vi "Configure Clock.vi"(7 "Interpolation":u16=1, 8 "error in (no error)":errorcluster, 9 "Rate of External Sample Clock (MHz)":u16=60 min=60 max=100 step=1, 10 "Clock Select":u32, 11 "FPGA VI Reference In":refnum<k20>) -> (0 "error out":errorcluster, 1 "User Command Error":u16, 2 "Successfully Configured?":bool, 3 "FPGA VI Reference Out":refnum<k20>, 4 "Sampling Rate":dbl)   [LabVIEW 2020]
uses:
  Controls/User Command.ctl
  <vilib>/Utility/error.llb/Error Cluster From Error Code.vi
  <vilib>/rvi/errors/niLvFpgaAdjustHostInterfaceError.vi
  <vilib>/rvi/interface/nirviReadWriteControl/nirviReadWriteControl.xnode
  NiFpgaLv.dll
  <vilib>/rvi/interface/Simulation/niFpgaSimulationCallBeginRW.vi
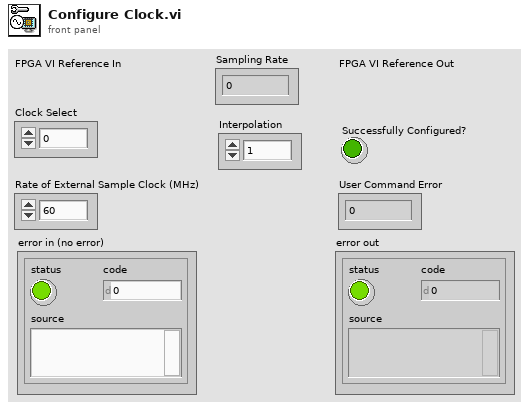
[diagram p1: front panel]
types:
  T1 = typedef "User Command.ctl" = u16
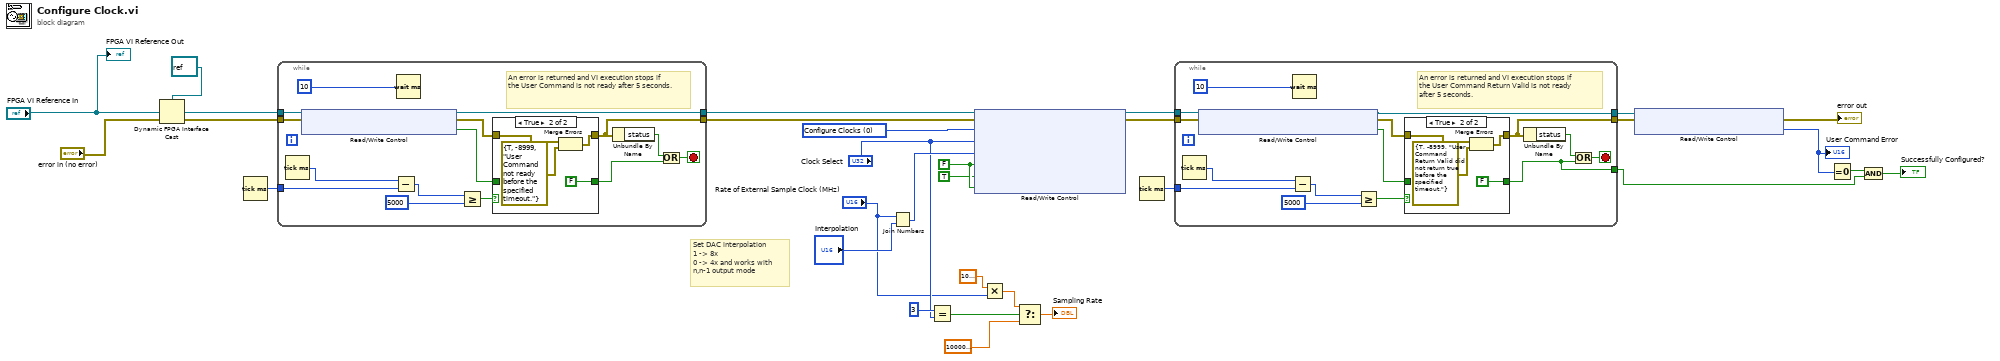
[diagram p0: block diagram]
diagram:
  w24 = FALSE ("IO Module\\User Command Valid")
  w25 = T1 0 items=["Reintialize"=65535, "Get CLIP Version"=65520, "SPI Write Verify"=65026, "SPI Write"=65025, "SPI Read"=65024, "I2C Write"=64769, "I2C Read"=64768, "Configure Clocks"=0]
  # "Set DAC interpolation \n1 -> 8x\n0 -> 4x and works with \nn,n-1 output mode"
  n1 = Dynamic FPGA Interface Cast(Session In=refnum<k20> refnum ("Refnum in"), Type="FPGA VI Reference In") -> (Session Out=w28:refnum<k20>)
  n2 = Tick Count (ms)() -> (millisecond timer value=w27:u32)
  n3 = while {
    tunnel: "error in (no error)" -> [w38]
    tunnel: [w42] -> w20
    tunnel: w28 -> [w37]
    tunnel: w27 -> [w33]
    tunnel: [w31] -> w26
    stop <- w40 stop-if-true
    # "An error is returned and VI execution stops if the User Command is not ready after 5 seconds."
    n4 = Tick Count (ms)() -> (millisecond timer value=w34:u32)
    n5 = xnode "Read/Write Control"("FPGA VI Reference In"=w37, "error in"=w38) -> ("FPGA VI Reference Out"=w31:refnum<k20>, "error out"=w35:errorcluster, "IO Module\\User Command Ready"=w36:bool)
    n6 = Subtract(x=w34, y=w33) -> (x-y=w32:u32)
    n7 = Wait (ms)(milliseconds to wait=u32 10) -> ()  [unwired: 1 out]
    n8 = Greater Or Equal?(x=w32, y=u32 5000) -> (x >= y?=w43:bool)
    n9 = case shown="True" w43 {
      tunnel: [w47 FALSE ("Configured?")] -> w39
      tunnel: w36 -> [w47 _]
      tunnel: [w46 w50] -> w42
      tunnel: w35 -> [w46 w48]
      frame False {
      }
      frame True {
        n10 = Merge Errors(w48, errorcluster {"status"=TRUE, "code"=-8999, "source"="User Command not ready before the specified timeout."} ("error in")) -> (w50:errorcluster)
      }
    }
    n11 = Unbundle By Name(w42) -> ("status"=w41:bool)
    n12 = Or(x=w41, y=w39) -> (x .or. y?=w40:bool)
  }
  n13 = Join Numbers(hi="Rate of External Sample Clock (MHz)", lo="Interpolation") -> ((hi.lo)=w21:u32)
  n14 = Equal?(x=u16 3, y="Clock Select") -> (x = y?=w8:bool)
  n15 = xnode "Read/Write Control"("FPGA VI Reference In"=w26, "error in"=w20, "IO Module\\User Command"=w25, "IO Module\\User Command Arg 0"="Clock Select", "IO Module\\User Command Arg 1"=w21, "IO Module\\User Command Valid"=w24, "IO Module\\User Command Valid"=TRUE ("IO Module\\User Command Valid"), "IO Module\\User Command Valid"=w24) -> ("FPGA VI Reference Out"=w18:refnum<k20>, "error out"=w17:errorcluster)
  n16 = Multiply(x=1000000.0 ("Sample Rate"), y="Rate of External Sample Clock (MHz)") -> (x*y=w5:dbl)
  n17 = Select(t=w5, s=w8, f=100000000.0 ("Sample Rate")) -> (s? t:f=→"Sampling Rate":dbl)
  n18 = Tick Count (ms)() -> (millisecond timer value=w19:u32)
  n19 = while {
    tunnel: w17 -> [w60]
    tunnel: [w63] -> w11
    tunnel: w18 -> [w59]
    tunnel: w19 -> [w55]
    tunnel: [w53] -> w16
    tunnel: [w52] -> w13
    stop <- w61 stop-if-true
    # "An error is returned and VI execution stops if the User Command Return Valid is not ready after 5 seconds."
    n20 = Tick Count (ms)() -> (millisecond timer value=w56:u32)
    n21 = xnode "Read/Write Control"("FPGA VI Reference In"=w59, "error in"=w60) -> ("FPGA VI Reference Out"=w53:refnum<k20>, "error out"=w57:errorcluster, "IO Module\\User Command Return Valid"=w58:bool)
    n22 = Subtract(x=w56, y=w55) -> (x-y=w54:u32)
    n23 = Wait (ms)(milliseconds to wait=u32 10) -> ()  [unwired: 1 out]
    n24 = Greater Or Equal?(x=w54, y=u32 5000) -> (x >= y?=w64:bool)
    n25 = case shown="True" w64 {
      tunnel: [w68 FALSE ("Configured?")] -> w52
      tunnel: w58 -> [w68 _]
      tunnel: [w67 w71] -> w63
      tunnel: w57 -> [w67 w69]
      frame False {
      }
      frame True {
        n26 = Merge Errors(w69, errorcluster {"status"=TRUE, "code"=-8999, "source"="User Command Return Valid did not return true before the specified timeout."} ("error in")) -> (w71:errorcluster)
      }
    }
    n27 = Unbundle By Name(w63) -> ("status"=w62:bool)
    n28 = Or(x=w62, y=w52) -> (x .or. y?=w61:bool)
  }
  n29 = xnode "Read/Write Control"("FPGA VI Reference In"=w16, "error in"=w11) -> ("error out"=→"error out":errorcluster, "IO Module\\User Command Error"=w15:u16)  [unwired: 1 out]
  "User Command Error" <- w15
  n30 = Equal To 0?(x=w15) -> (x = 0?=w14:bool)
  n31 = And(x=w14, y=w13) -> (x .and. y?=→"Successfully Configured?":bool)
  "FPGA VI Reference Out" <- "FPGA VI Reference In"
